vi "Natural Logarithm - RM.vi"(1 "Real Matrix A":T2) -> (0 "ln(A)":T1)   [LabVIEW 2020, in "NI_Matrix.lvlib"]
doc: "Computes the natural logarithm of the input matrix."
uses:
  NI_Matrix.lvlib
  RealMatrix.ctl
  ComplexMatrix.ctl
  Real Matrix Logarithm.vi
  NI_AALBase.lvlib
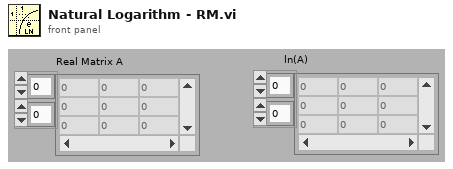
[diagram p1: front panel]
types:
  T1 = typedef "NI_Matrix.lvlib/ComplexMatrix.ctl" = cdb[][]
  T2 = typedef "NI_Matrix.lvlib/RealMatrix.ctl" = dbl[][]
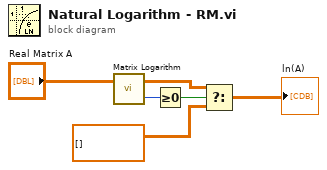
[diagram p0: block diagram]
diagram:
  n1 = call-poly "Matrix Logarithm.vi"("Input Matrix"="Real Matrix A") -> ("error"=w1:i32, "Matrix Logarithm"=w2:T1)  [unwired: 1 in]
  n2 = Greater Or Equal To 0?(x=w1) -> (x >= 0?=w6:bool)
  n3 = Select(t=w2, s=w6, f=T1 [] ("ln(A)")) -> (s? t:f=→"ln(A)":T1)
